vi "Enable Disable Enum to Enabled.vi"(1 "Disabled":T1(ring)) -> (0 "Enabled":bool)   [LabVIEW 2018]
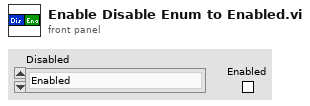
[diagram p1: front panel]
types:
  T1 = enum8{"Enabled", "Disabled", "Disabled and Grayed Out"}
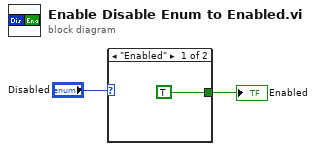
[diagram p0: block diagram]
diagram:
  n1 = case shown="\"Enabled\"" "Disabled" {
    tunnel: [TRUE _] -> w1
    frame "Enabled" {
    }
    frame Default {
    }
  }
  "Enabled" <- w1
